vi "PeekOpen.vi"(11 "RVCLibrary_Bug2 in":refnum<class "RVCLibrary_Bug2.lvclass">) -> (2 "node ref out":refnum<data-value>, 3 "RVCLibrary_Bug2 out":refnum<class "RVCLibrary_Bug2.lvclass">)   [LabVIEW 2013, in "RVCLibrary_Bug2.lvclass"]
uses:
  RVCLibrary_Bug2.lvclass
  <vilib>/robotics/Navigation/shared/MapNode/AbstractDstarNode/NI_Robotics_AbstractDstarNode.lvclass
  <vilib>/robotics/Navigation/shared/MapNode/AbstractMapNode/NI_Robotics_AbstractMapNode.lvclass
  RVCLibrary_Bug2.lvclass/RVCLibrary_Bug2.ctl
  <vilib>/robotics/Navigation/shared/Priority Queue/NI_Robotics_Priority Queue.lvclass
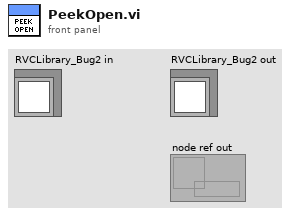
[diagram p1: front panel]
types:
  T1 = typedef "NI_Robotics_Priority Queue.lvclass/Open List Element.ctl" = cluster{"f":dbl, "g":dbl, "node Ref":refnum<data-value>}
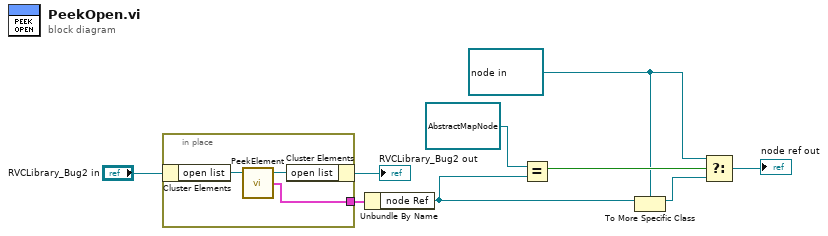
[diagram p0: block diagram]
diagram:
  w4 = refnum<data-value> refnum ("node ref out")
  n1 = in-place {
    in-place-border: [w10] -> w9
    n2 = in-place-cluster #1("RVCLibrary_Bug2 in") -> ("open list"=w12:refnum<class "NI_Robotics_Priority Queue.lvclass">)
    n3 = call <vilib>:"PeekElement.vi"("Astar Open List in"=w12) -> ("Open List Element"=w10:T1, "Astar Open List out"=w11:refnum<class "NI_Robotics_Priority Queue.lvclass">)  [unwired: 2 in, 1 out]
    n4 = in-place-cluster #1("open list"=w11) -> (→"RVCLibrary_Bug2 out":refnum<class "RVCLibrary_Bug2.lvclass">)
  }
  n5 = Unbundle By Name(w9) -> ("node Ref"=w8:refnum<data-value>)
  n6 = Equal?(x=refnum<data-value> refnum ("node Ref"), y=w8) -> (x = y?=w5:bool)
  n7 = To More Specific Class(target class=w4, reference=w8) -> (specific class reference=w7:refnum<data-value>)  [unwired: 1 in, 1 out]
  n8 = Select(t=w4, s=w5, f=w7) -> (s? t:f=→"node ref out":refnum<data-value>)
